vi "FFT.vi"(9 "FFT模式":enum16{"对称FFT", "单边FFT", "FFT功率"}(ring), 10 "window":T1 items=["矩形"=0, "Hanning"=1, "Hamming"=2, "Blackman-Harris"=3, "Exact Blackman"=4, "Blackman"=5, "Flat Top"=6, "4阶Blackman-Harris "=7, "7阶Blackman-Harris"=8, "Low Sidelobe"=9, "Blackman Nuttall"=11, "三角"=30, "Bartlett-Hanning"=31, "Bohman"=32, "Parzen"=33, "Welch"=34, "Kaiser"=60, "Dolph-Chebyshev"=61, "高斯"=62], 11 "输入X":dbl[](array[numeric])) -> (3 "FFT输出":dbl[](array[numeric]))   [LabVIEW 2014]
uses:
  <vilib>/Analysis/4window.llb/windowTd.ctl
  <vilib>/measure/maspectr.llb/FFT Spectrum (Mag-Phase) for 1 Chan.vi
  <vilib>/measure/maspectr.llb/FFT Power Spectrum and PSD for 1 Chan.vi
  <vilib>/measure/NI_MAPro.lvlib
  <vilib>/Analysis/NI_AALPro.lvlib
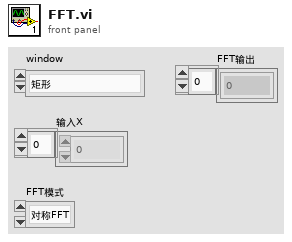
[diagram p1: front panel]
types:
  T1 = typedef "NI_AALPro.lvlib/windowTd.ctl" = u32
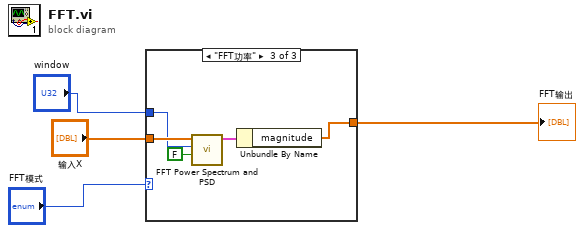
[diagram p0: block diagram]
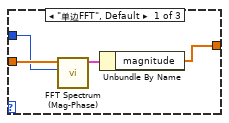
[diagram p2: hidden frame]
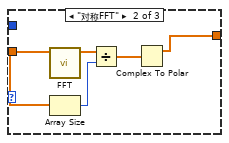
[diagram p3: hidden frame]
diagram:
  n1 = case shown="\"FFT功率\"" "FFT模式" {
    tunnel: "输入X" -> [w7 w10 w17]
    tunnel: [w6 w9 w16] -> w3
    tunnel: "window" -> [w5 _ w15]
    frame "单边FFT", Default {
      n2 = call-poly <vilib>:"FFT Spectrum (Mag-Phase).vi"("window"=w5, "time signal"=w7) -> ("magnitude"=w8:cluster{"f0":dbl, "df":dbl, "magnitude":dbl[]})  [unwired: 5 in, 4 out]
      n3 = Unbundle By Name(w8) -> ("magnitude"=w6:dbl[])
    }
    frame "对称FFT" {
      n4 = call-poly <vilib>:"FFT.vi"("X"=w10) -> ("FFT {X}"=w11:cdb[])  [unwired: 9 in, 1 out]
      n5 = Array Size(array=w10) -> (size(s)=w13:i32)
      n6 = Divide(x=w11, y=w13) -> (x/y=w12:cdb[])
      n7 = Complex To Polar(r * e^(i*theta)=w12) -> (r=w9:dbl[])  [unwired: 1 out]
    }
    frame "FFT功率" {
      n8 = call-poly <vilib>:"FFT Power Spectrum and PSD.vi"("dB On (F)"=FALSE, "window"=w15, "time signal"=w17) -> ("Power Spectrum / PSD"=w18:cluster{"f0":dbl, "df":dbl, "magnitude":dbl[]})  [unwired: 5 in, 3 out]
      n9 = Unbundle By Name(w18) -> ("magnitude"=w16:dbl[])
    }
  }
  "FFT输出" <- w3
